vi "setCommand.vi"(8 "error in (no error)":errorcluster, 10 "command":T1=enum."stop sweep", 11 "Generator in":refnum<class "Generator.lvclass">) -> (0 "error out":errorcluster, 3 "Generator out":refnum<class "Generator.lvclass">)   [LabVIEW 2019, in "Generator.lvclass"]
uses:
  Generator.lvclass
  Generator.lvclass/Generator.ctl
  typedefs/Generator.Command--enum.ctl
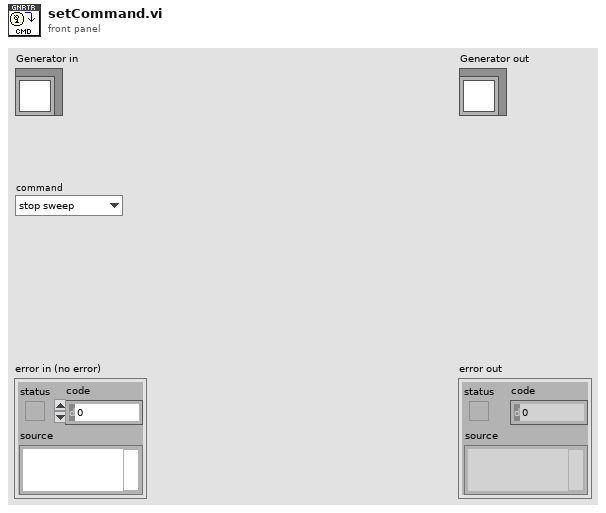
[diagram p1: front panel]
types:
  T1 = typedef "Generator.lvclass/Generator.Command--enum.ctl" = enum16{"start", "stop", "start sweep", "stop sweep"}
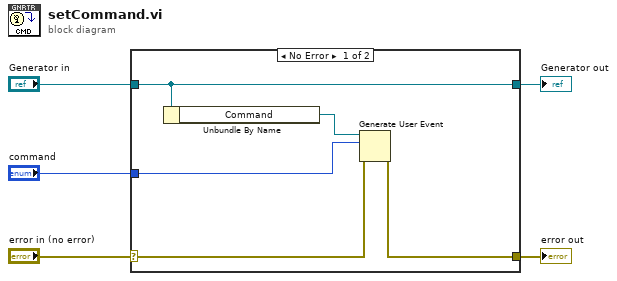
[diagram p0: block diagram]
diagram:
  n1 = case shown="No Error" "error in (no error)" {
    selector: "error in (no error)" -> [w10 w11]
    tunnel: [w9 w11] -> w4
    tunnel: [w8 w12] -> w2
    tunnel: "Generator in" -> [w8 w12]
    tunnel: "command" -> [w6 _]
    frame No Error {
      n2 = Unbundle By Name(w8) -> ("Command"=w7:refnum<user-event>)
      n3 = Generate User Event(user event=w7, event data cluster=w6, error in=w10) -> (error out=w9:errorcluster)  [unwired: 1 in, 1 out]
    }
    frame Error {
    }
  }
  "error out" <- w4
  "Generator out" <- w2
